vi "Check Movement.vi"(11 "MAS ACTOR in":refnum<class "MAS ACTOR.lvclass">=refnum) -> (3 "MAS ACTOR out":refnum<class "MAS ACTOR.lvclass">)   [LabVIEW 2022 SP3, in "MAS.lvlib" / "MAS ACTOR.lvclass"]
uses:
  MAS ACTOR.lvclass
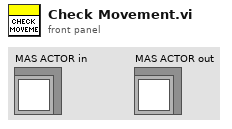
[diagram p1: front panel]
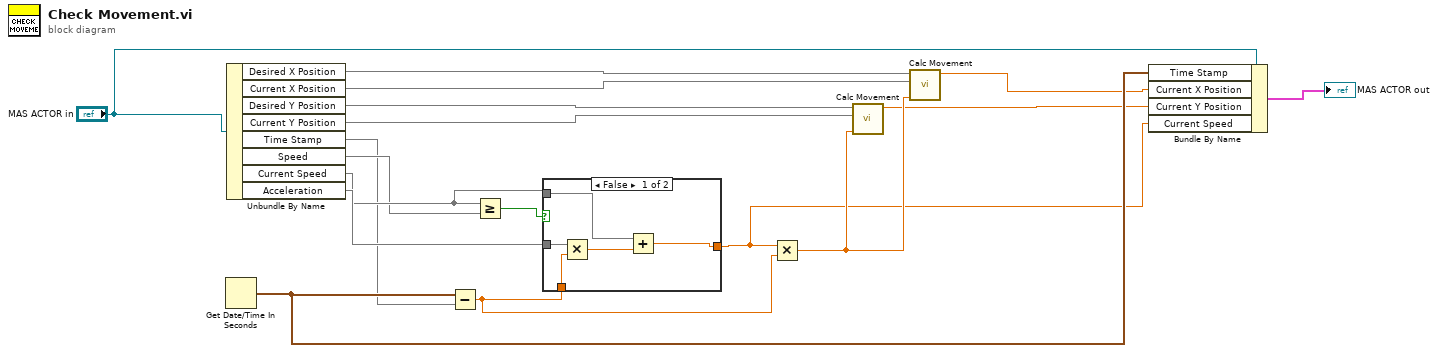
[diagram p0: block diagram]
diagram:
  n1 = Get Date/Time In Seconds() -> (seconds since 1Jan1904=w11:timestamp)
  n2 = Unbundle By Name("MAS ACTOR in") -> ("Desired X Position"=w4, "Current X Position"=w5, "Desired Y Position"=w6, "Current Y Position"=w7, "Time Stamp"=w10, "Speed"=w12, "Current Speed"=w14, "Acceleration"=w16)
  n3 = Subtract(x=w11, y=w10) -> (x-y=w15:dbl)
  n4 = Greater Or Equal?(x=w14, y=w12) -> (x >= y?=w13:bool)
  n5 = case shown="False" w13 {
    tunnel: [w18 w23] -> w1
    tunnel: w14 -> [w19 w23]
    tunnel: w15 -> [w22 _]
    tunnel: w16 -> [w21 _]
    frame False {
      n6 = Multiply(x=w21, y=w22) -> (x*y=w20:dbl)
      n7 = Add(x=w19, y=w20) -> (x+y=w18:dbl)
    }
    frame True {
    }
  }
  n8 = Multiply(x=w1, y=w15) -> (x*y=w17:dbl)
  n9 = call "Calc Movement.vi"("New Distance"=w17, "Current"=w7, "Desired"=w6) -> ("New Current"=w9:dbl)  [unwired: 8 in]
  n10 = call "Calc Movement.vi"("New Distance"=w17, "Current"=w5, "Desired"=w4) -> ("New Current"=w8:dbl)  [unwired: 8 in]
  n11 = Bundle By Name(cluster="MAS ACTOR in", "Time Stamp"=w11, "Current X Position"=w8, "Current Y Position"=w9, "Current Speed"=w1) -> (→"MAS ACTOR out":cluster{})
